vi "8P_Clone.vi"(0 "Single 8HP":T1) -> (2 "DAQ Error":errorcluster, 3 "All samples out":sgl[][](array[numeric]), 4 "Ch No":i16[](array[numeric]), 5 "Index":i32[](array[numeric]), 6 "Sampling Rate Hz":dbl)   [LabVIEW 2020]
doc: "Use this plug-in with the Nathan 7609 data acquisition system"
uses:
  Device ID port info.ctl
  8HP/ctls/8HP_Cmd (USB).ctl
  ctls/Cmd.ctl
  Globals/Meas_global.vi
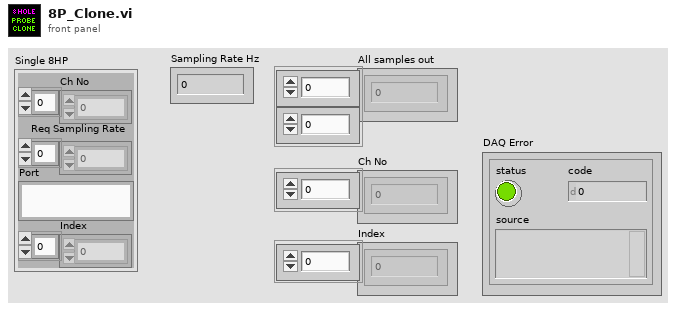
[diagram p1: front panel]
types:
  T1 = typedef "Device ID port info.ctl" = cluster{"Ch No":i16[], "Req Sampling Rate":dbl[], "Port":string, "Index":i32[]}
  T2 = typedef "Trigger_Mode.ctl" = enum16{"Free Running", "Start on Trigger", "Trigger Every Block", "Trigger Every Sample"}
  T3 = typedef "8HP_Cmd (USB).ctl" = string
  T4 = typedef "Cmd.ctl" = string
  T5 = typedef "Rendezvous RefNum" = refnum<k1>
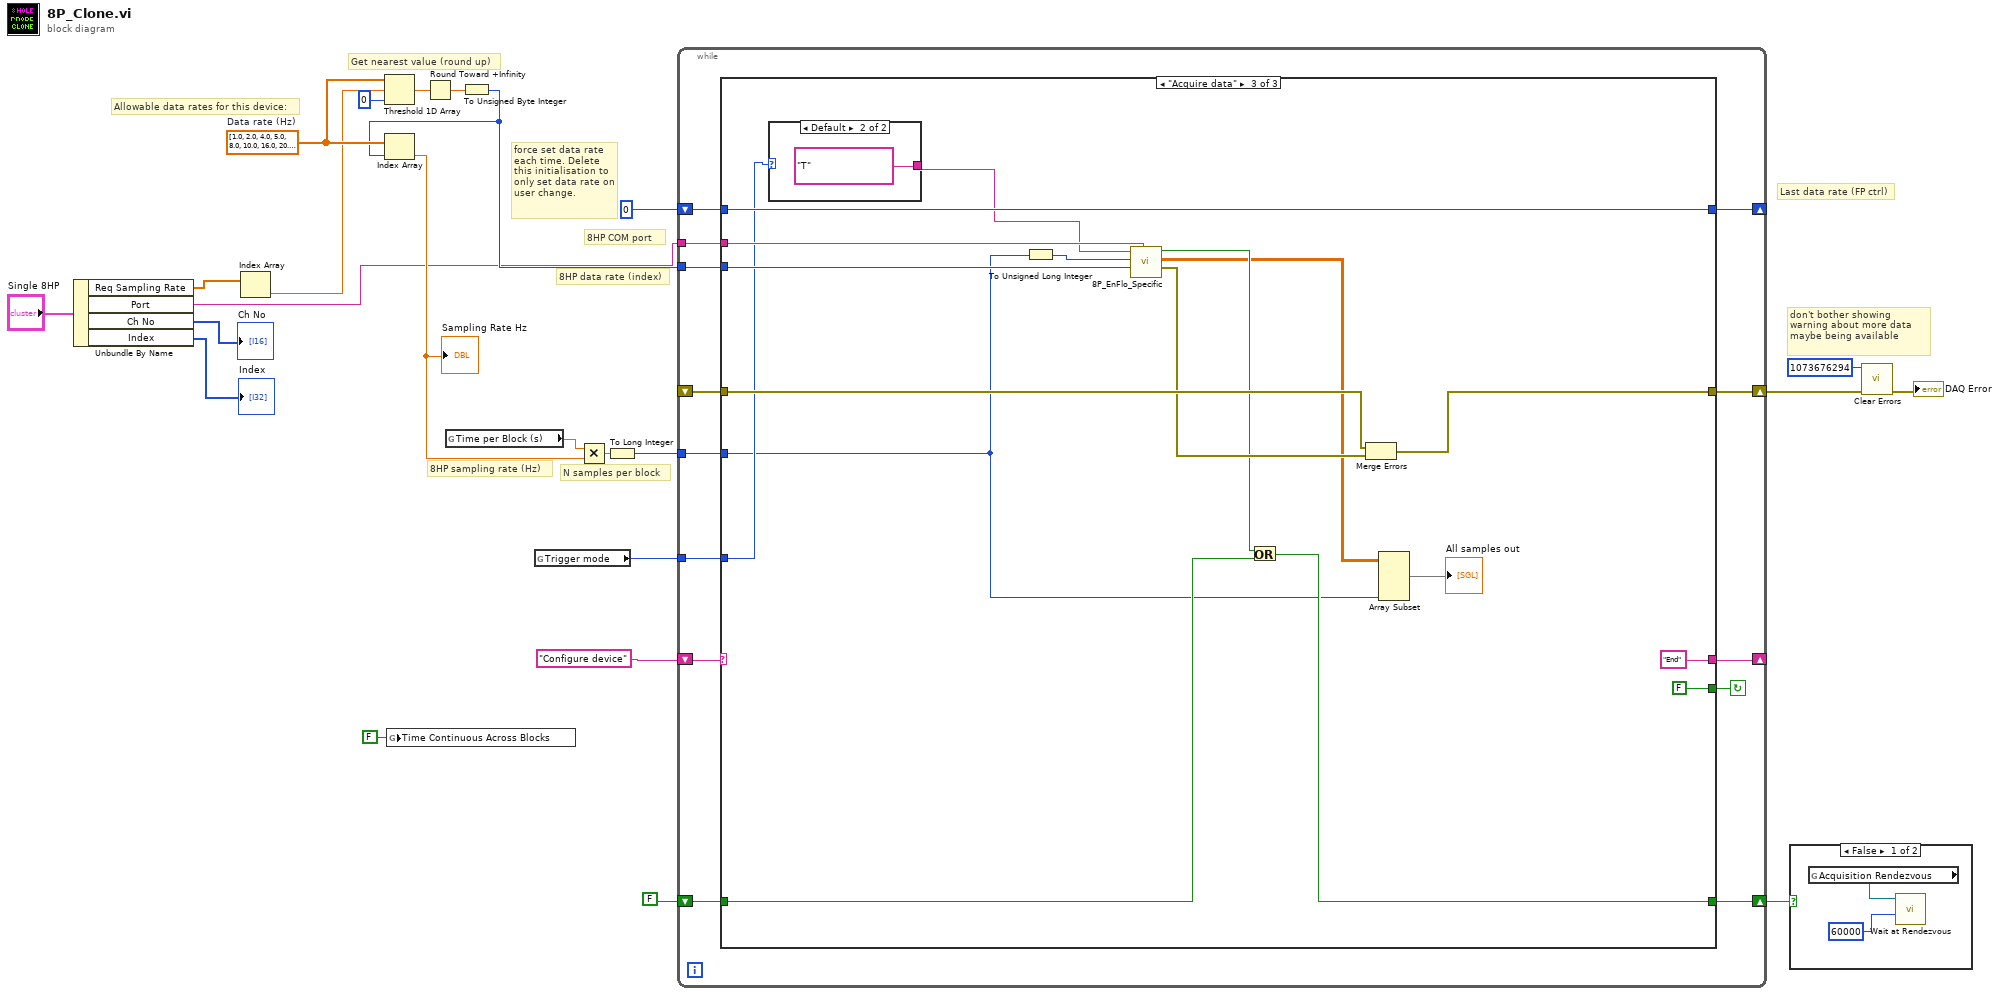
[diagram p0: block diagram]
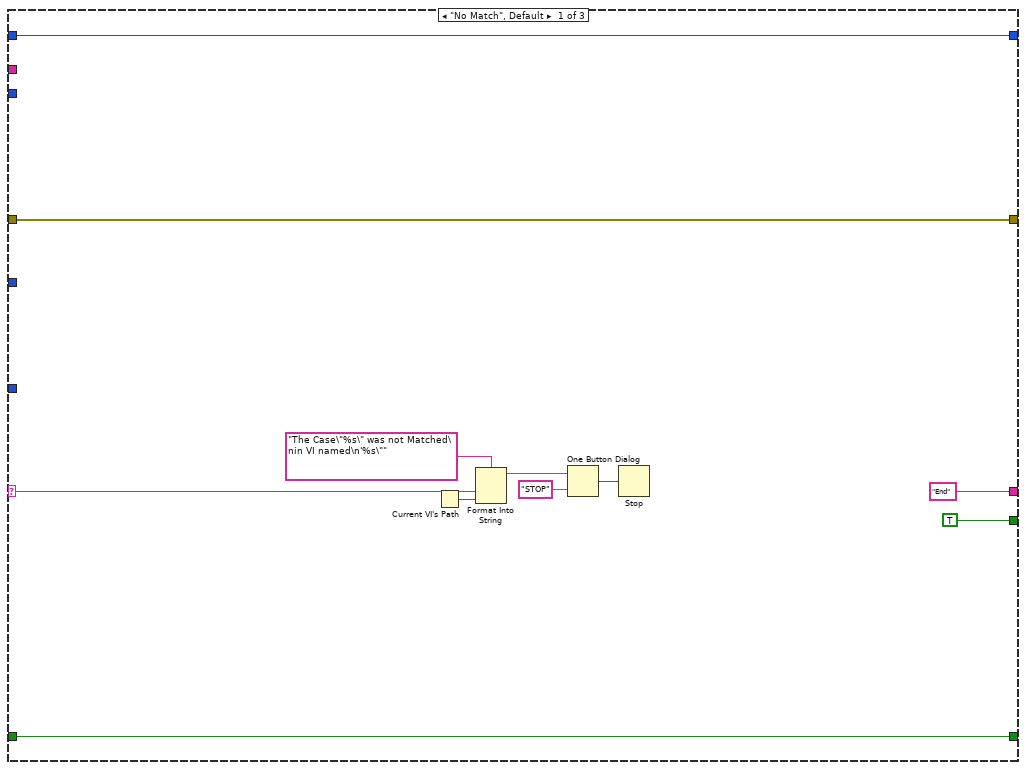
[diagram p3: hidden frame]
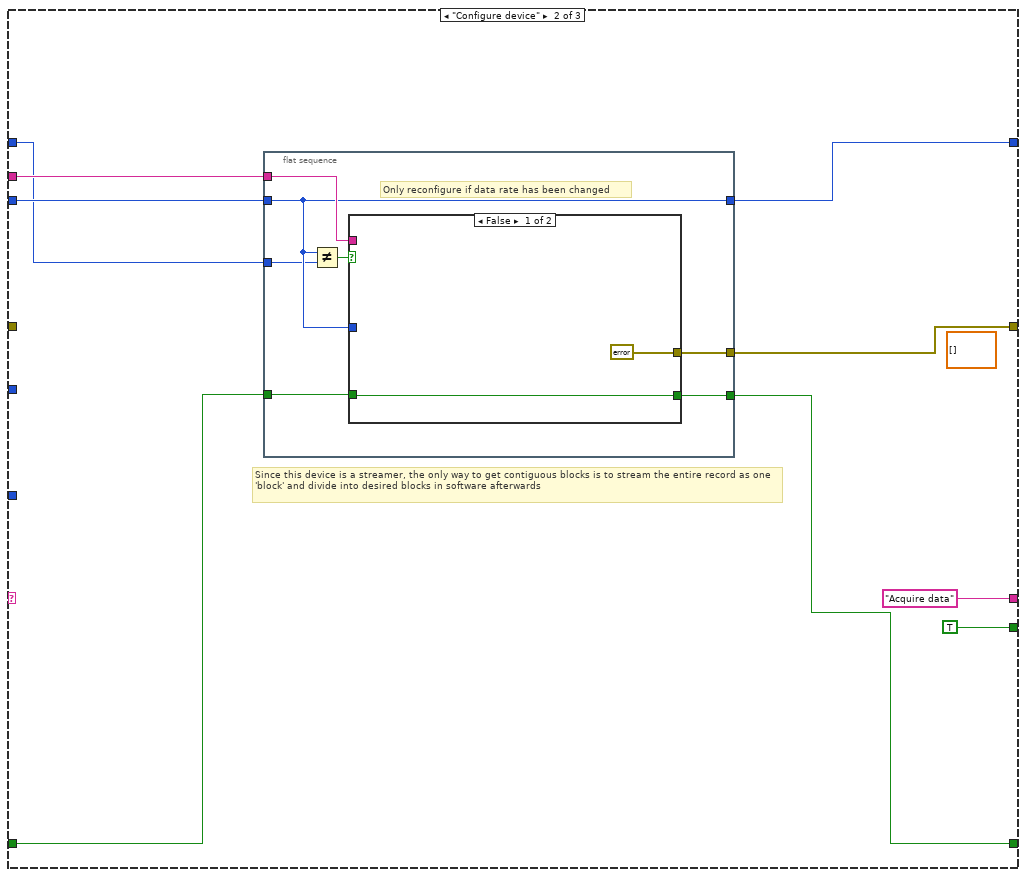
[diagram p4: hidden frame]
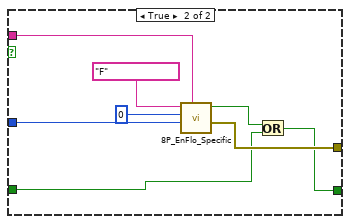
[diagram p5: hidden frame]
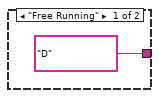
[diagram p6: hidden frame]
diagram:
  w17 = dbl[] [1.0, 2.0, 4.0, 5.0, 8.0, 10.0, 16.0, 20.0, 25.0, 32.0, 40.0, 50.0, 64.0, 80.0, 100.0, 125.0, 160.0, 200.0, 250.0, 320.0, 400.0, 500.0, 625.0, 800.0, 1000.0]  # Data rate (Hz)
  # "N samples per block"
  # "8HP sampling rate (Hz)"
  # "8HP COM port"
  # "8HP data rate (index)"
  # "Allowable data rates for this device:"
  # "Get nearest value (round up)"
  # "force set data rate each time. Delete this initialisation to only set data rate on user change."
  # "Last data rate (FP ctrl)"
  # "don't bother showing warning about more data maybe being available"
  n1 = Unbundle By Name("Single 8HP") -> ("Req Sampling Rate"=w8:dbl[], "Port"=w9:string, "Ch No"=→"Ch No":i16[], "Index"=→"Index":i32[])
  n2 = Index Array(array=w8) -> (element=w7:dbl)  [unwired: 1 in]
  n3 = Threshold 1D Array(1:0 ("start index (0)"), 2:w7, 3:w17) -> (0:w18:dbl)
  n4 = global write "Meas_global.vi" "Time Continuous Across Blocks"(FALSE ("Time Continuous Across Blocks")) -> ()
  n5 = Round Toward +Infinity(x=w18) -> (ceil(x): smallest int >= x=w16:dbl)
  n6 = global read "Meas_global.vi" "Time per Block (s)"() -> (w15:dbl)
  n7 = To Unsigned Byte Integer(number=w16) -> (unsigned 8bit integer=w11:u8)
  n8 = Index Array(array=w17, index=w11) -> (element=w12:dbl)
  "Sampling Rate Hz" <- w12
  n9 = global read "Meas_global.vi" "Trigger mode"() -> (w4:T2)
  n10 = Multiply(x=w15, y=w12) -> (x*y=w14:dbl)
  n11 = To Long Integer(number=w14) -> (32bit integer=w13:i32)
  n12 = while {
    shift-left: "Configure device" -> [w37]
    shift-right: [w32] -> _
    tunnel: w13 -> [w36]
    shift-right: [w33] -> w21
    shift-left: _ -> [w34]
    tunnel: w9 -> [w31]
    tunnel: w11 -> [w30]
    shift-right: [w29] -> _
    shift-left: u8 0 ("Pressure data rate (Hz)") -> [w28]
    tunnel: w4 -> [w27]
    shift-right: [w25] -> w2
    shift-left: FALSE -> [w26]
    stop <- w35 continue-if-true
    n13 = case shown="\"Acquire data\"" w37 {
      selector: w37 -> [w41 _ _]
      tunnel: ["End" "Acquire data" ("f") "End"] -> w32
      tunnel: w36 -> [_ _ w76]
      tunnel: [TRUE TRUE FALSE] -> w35
      tunnel: w34 -> [w40 _ w89]
      tunnel: [w40 w56 w88] -> w33
      tunnel: w31 -> [_ w54 w87]
      tunnel: w30 -> [_ w53 w86]
      tunnel: [w39 w52 w85] -> w29
      tunnel: w28 -> [w39 w51 w85]
      tunnel: w27 -> [_ _ w83]
      tunnel: w26 -> [w38 w50 w82]
      tunnel: [w38 w49 w81] -> w25
      frame "No Match", Default {
        n14 = Current VI's Path() -> (path=w44:path)
        n15 = Format Into String(format string="The Case\"%s\" was not Matched\nin VI named\n'%s\"" ("Format String"), w41, w44) -> (resulting string=w47:string)  [unwired: 2 in, 1 out]
        n16 = One Button Dialog(message=w47, button name ("OK")="STOP") -> (true=w45:bool)
        n17 = Stop(stop? (T)=w45) -> ()
      }
      frame "Configure device" {
        (unwired) sgl[][] [] ("Channel volts")
        # "Since this device is a streamer, the only way to get contiguous blocks is to stream the entire record as one 'block' and divide into desired blocks in software afterwards"
        n18 = flat-sequence {
          tunnel: w54 -> [w63]
          tunnel: w53 -> [w61]
          tunnel: w51 -> [w60]
          tunnel: w50 -> [w59]
          tunnel: [w64] -> w56
          tunnel: [w61] -> w52
          tunnel: [w58] -> w49
          frame #0 {
            # "Only reconfigure if data rate has been changed"
            n19 = Not Equal?(x=w61, y=w60) -> (x != y?=w62:bool)
            n20 = case shown="False" w62 {
              tunnel: [errorcluster {"status"=FALSE, "code"=0, "source"=""} ("error IO") w71] -> w64
              tunnel: w63 -> [_ w70]
              tunnel: w61 -> [_ w72]
              tunnel: w59 -> [w65 w68]
              tunnel: [w65 w67] -> w58
              frame False {
              }
              frame True {
                n21 = call "8P_EnFlo_Specific.vi"("COM port"=w70, "Data rate (Hz)"=w72, "N samples"=u32 0, "Command"=T3 "F") -> ("Error"=w71:errorcluster, "Rendezvous Out"=w69:bool)  [unwired: 2 in, 2 out]
                n22 = Or(x=w69, y=w68) -> (x .or. y?=w67:bool)
              }
            }
          }
        }
      }
      frame "Acquire data" {
        n23 = case shown="Default" w83 {
          tunnel: [T4 "D" ("Combo Box") T4 "T" ("Combo Box")] -> w84
          frame "Free Running" {
          }
          frame Default {
          }
        }
        n24 = To Unsigned Long Integer(number=w76) -> (unsigned 32bit integer=w79:u32)
        n25 = call "8P_EnFlo_Specific.vi"("COM port"=w87, "Data rate (Hz)"=w86, "N samples"=w79, "Command"=w84) -> ("Error"=w80:errorcluster, "All samples out"=w77:sgl[][], "Rendezvous Out"=w78:bool)  [unwired: 2 in, 1 out]
        n26 = Or(x=w78, y=w82) -> (x .or. y?=w81:bool)
        n27 = Merge Errors(w89, w80) -> (w88:errorcluster)
        n28 = Array Subset(array=w77, length (col)=w76) -> (→"All samples out":sgl[][])  [unwired: 3 in]
      }
    }
  }
  n29 = case shown="False" w2 {
    frame False {
      n30 = global read "Meas_global.vi" "Acquisition Rendezvous"() -> (w95:T5)
      n31 = call <vilib>:"Wait at Rendezvous.vi"("ms timeout (-1)"=60000, "rendezvous"=w95) -> ()  [unwired: 3 in, 3 out]
    }
    frame True {
    }
  }
  n32 = call <vilib>:"Clear Errors.vi"("error in (no error)"=w21, "specific error code to clear (0: all)"=1073676294) -> ("error out"=→"DAQ Error":errorcluster)  [unwired: 4 in, 1 out]
